vi "Overlay.vi"(8 "error in (no error)":errorcluster, 10 "Image In":T1, 11 "Overlay Base in":refnum<class "Analyze Results Distanz.lvclass">) -> (0 "error out":errorcluster, 2 "Image out":T1, 3 "Overlay Base out":refnum<class "Analyze Results Distanz.lvclass">)   [LabVIEW 2014, in "Analyze Results Distanz.lvclass"]
uses:
  Analyze Results Distanz.lvclass
  <vilib>/vision/Image Controls.llb/IMAQ Image.ctl
  Results Base/Analyze Results Base.lvclass/Analyze Results Base.ctl
  Analyze Results Distanz.lvclass/Analyze Results Distanz.ctl
  Results Base/Read Overlay_.vi
  Results Base/Read Overlay colors.vi
  Results Base/Read Font, Size & Style.vi
  Results Base/Analyze Results Base.lvclass
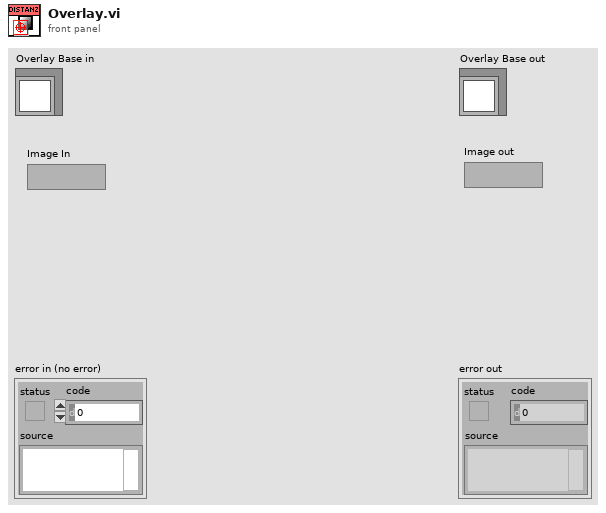
[diagram p1: front panel]
types:
  T1 = typedef "IMAQ Image.ctl" = refnum<image>
  T2 = cluster{"Desired Font (Application)":enum16{"User-specified Font", "Application Font", "System Font", "Dialog Font"}, "[User-specified Font]":cluster{"Font Name":string, "Size":i16, "Strikeout?":bool, "Italic?":bool, "Underline?":bool, "Outline?":bool, "Shadow?":bool, "Bold?":bool, "Rotation Angle":dbl}, "Horizontal Alignment":i16, "Vertical Alignment":i16}
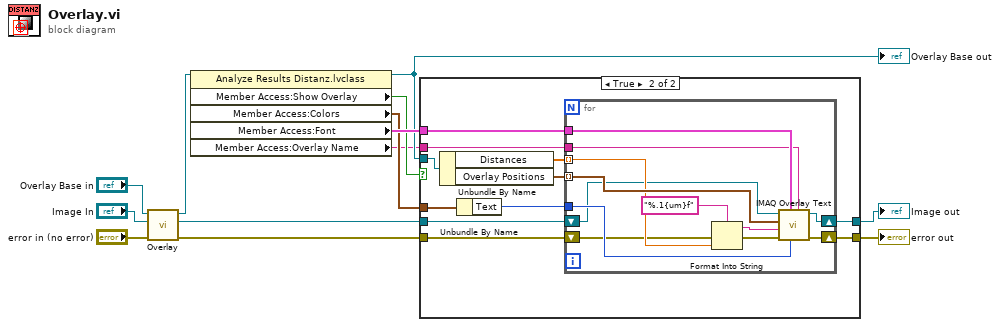
[diagram p0: block diagram]
diagram:
  n1 = call-parent "Overlay.vi"("error in (no error)"="error in (no error)", "Image In"="Image In", "Overlay Base in"="Overlay Base in") -> ("error out"=w3:errorcluster, "Image out"=w5:T1, "Overlay Base out"=w10:refnum<class "Analyze Results Distanz.lvclass">)  [unwired: 6 in]
  n2 = property class="Analyze Results Distanz.lvclass"(reference=w10) -> (reference out=w6:refnum<class "Analyze Results Distanz.lvclass">, "Member Access:Show Overlay"=w7:bool, "Member Access:Colors"=w8:cluster{"Border":u32, "Text":u32}, "Member Access:Font"=w9:T2, "Member Access:Overlay Name"=w1:string)  [unwired: 1 in, 1 out]
  "Overlay Base out" <- w6
  n3 = case shown="True" w7 {
    tunnel: w6 -> [_ w26]
    tunnel: w9 -> [_ w25]
    tunnel: w8 -> [_ w22]
    tunnel: w5 -> [w15 w20]
    tunnel: [w15 w19] -> w4
    tunnel: w3 -> [w14 w18]
    tunnel: [w14 w17] -> w2
    tunnel: w1 -> [_ w16]
    frame False {
    }
    frame True {
      n4 = Unbundle By Name(w26) -> ("Distances"=w23:dbl[unit][], "Overlay Positions"=w24:cluster{"x":i16, "y":i16}[])
      n5 = Unbundle By Name(w22) -> ("Text"=w21:u32)
      n6 = for {
        tunnel: w25 -> [w38]
        tunnel: w24 -> [w37] mode=indexing
        tunnel: w23 -> [w36] mode=indexing
        tunnel: w21 -> [w33]
        shift-right: [w31] -> w19
        shift-left: w20 -> [w32]
        shift-right: [w30] -> w17
        shift-left: w18 -> [w29]
        tunnel: w16 -> [w27]
        n7 = Format Into String(format string="%.1{um}f", error in=w29, w36) -> (resulting string=w35:string, error out=w28:errorcluster)  [unwired: 1 in]
        n8 = call "IMAQ Overlay Text"("Group"=w27, "Text Color (black)"=w33, "Font, Size & Style"=w38, "error in (no error)"=w28, "String"=w35, "Origin"=w37, "Image"=w32) -> ("error out"=w30:errorcluster, "Image Out"=w31:T1)  [unwired: 3 in]
      }
    }
  }
  "error out" <- w2
  "Image out" <- w4
